vi "DisplayLeg.vi"(4 "Init?":bool, 6 "ClosePt":dbl[](array[numeric]), 7 "Field Force":dbl[](array[numeric]), 8 "AnkleTraj":dbl[][](array[numeric]), 9 "CablePos":cluster{"PointInGCS":dbl[][]}[](array[cluster]), 10 "Joint Coord in GCS":dbl[][](array[numeric]), 11 "3D graph in":refnum<k7>) -> (3 "3D graph out":refnum<k7>)   [LabVIEW 2014]
uses:
  <vilib>/Platform/NI_3dgraph.lvlib
  <vilib>/ptbypt/NI_PtbyPt.lvlib
panel:
  in  "sample length":i32=100
  out "LastPlotNum":i32=1
  out "error out":errorcluster
  in  "error in (no error)":errorcluster
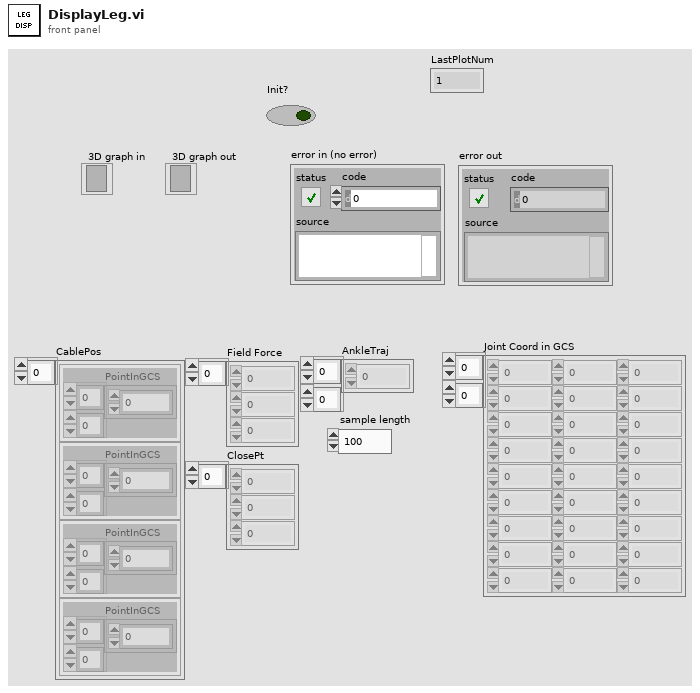
[diagram p1: front panel]
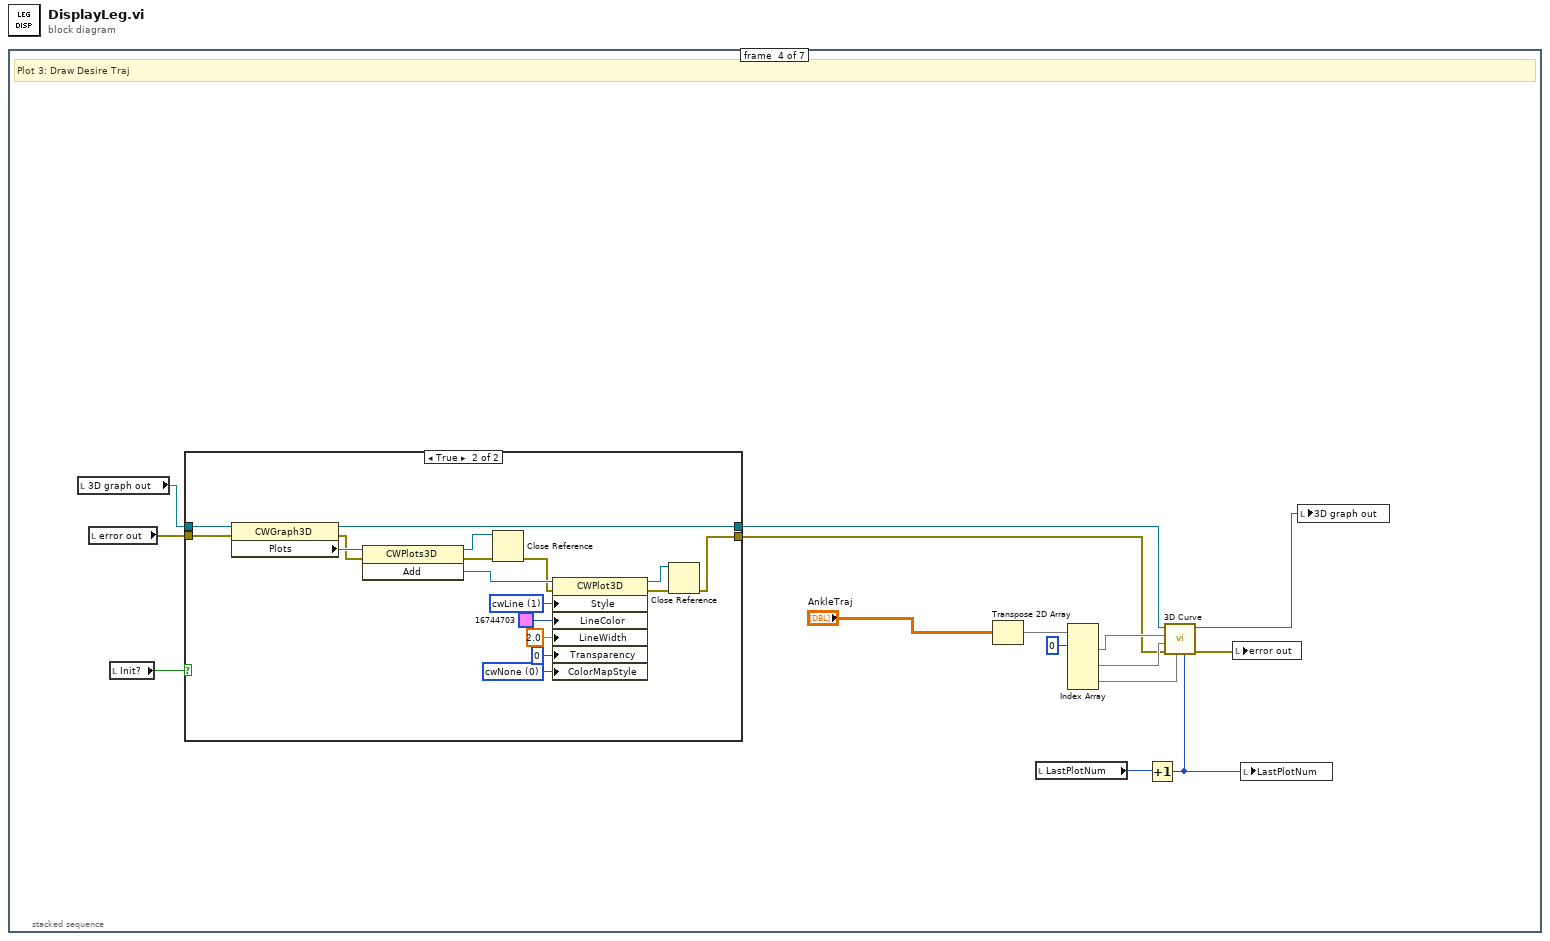
[diagram p0: block diagram]
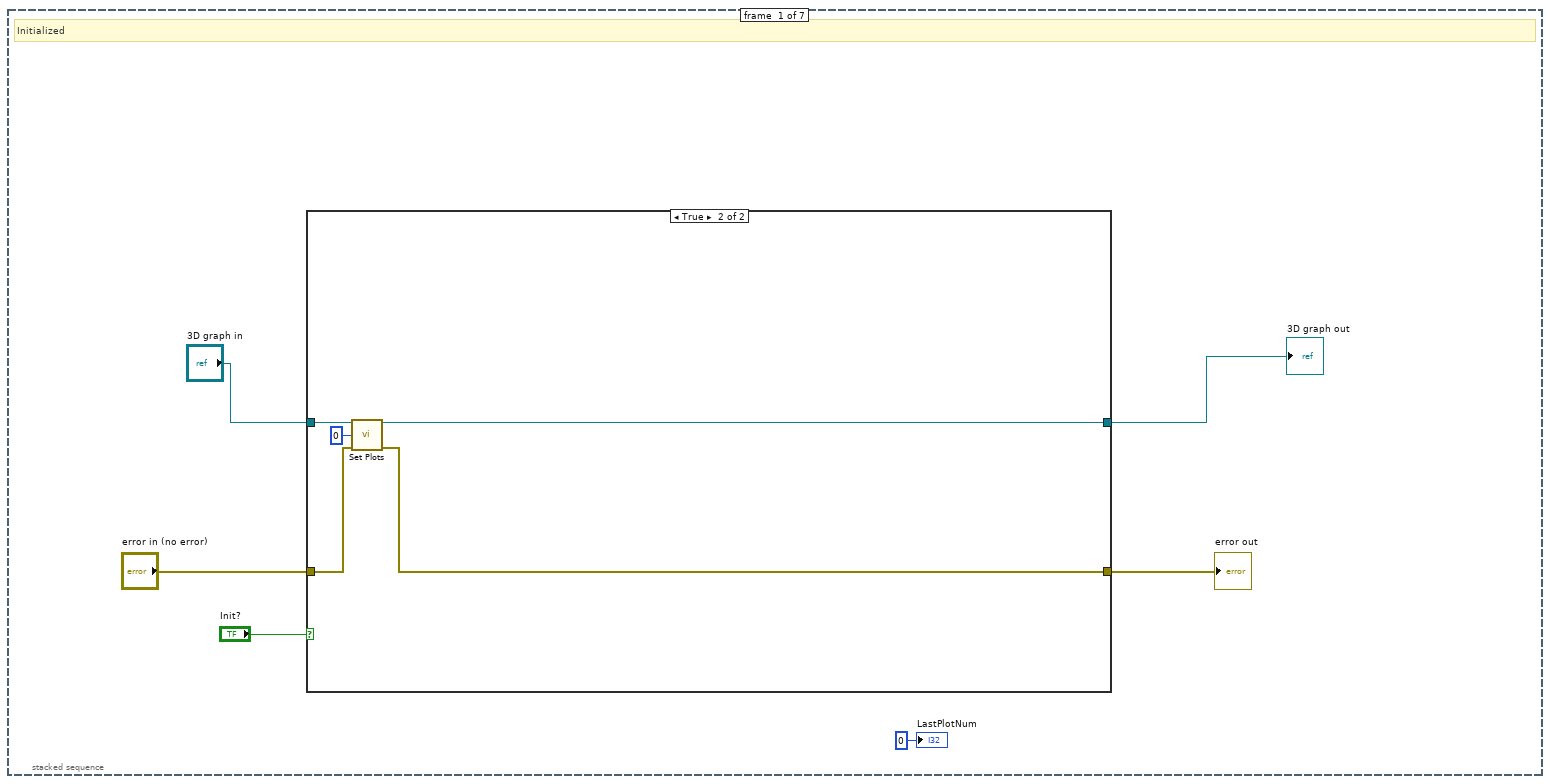
[diagram p2: hidden frame]
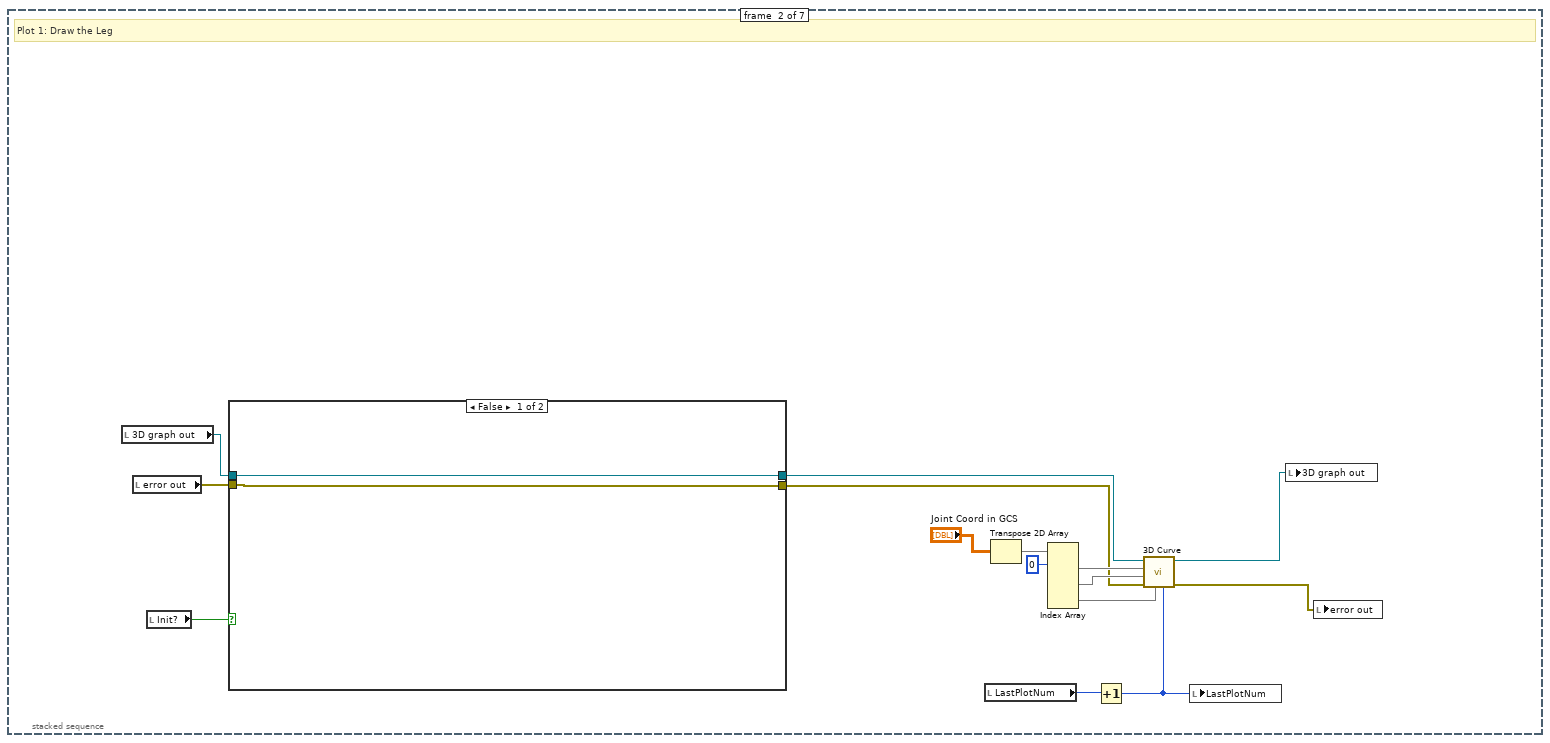
[diagram p4: hidden frame]
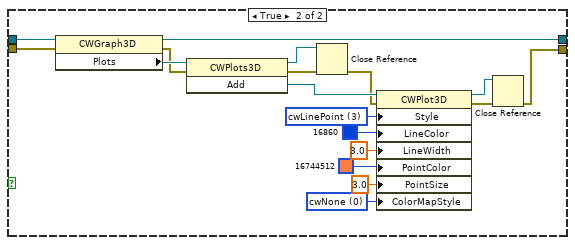
[diagram p5: hidden frame]
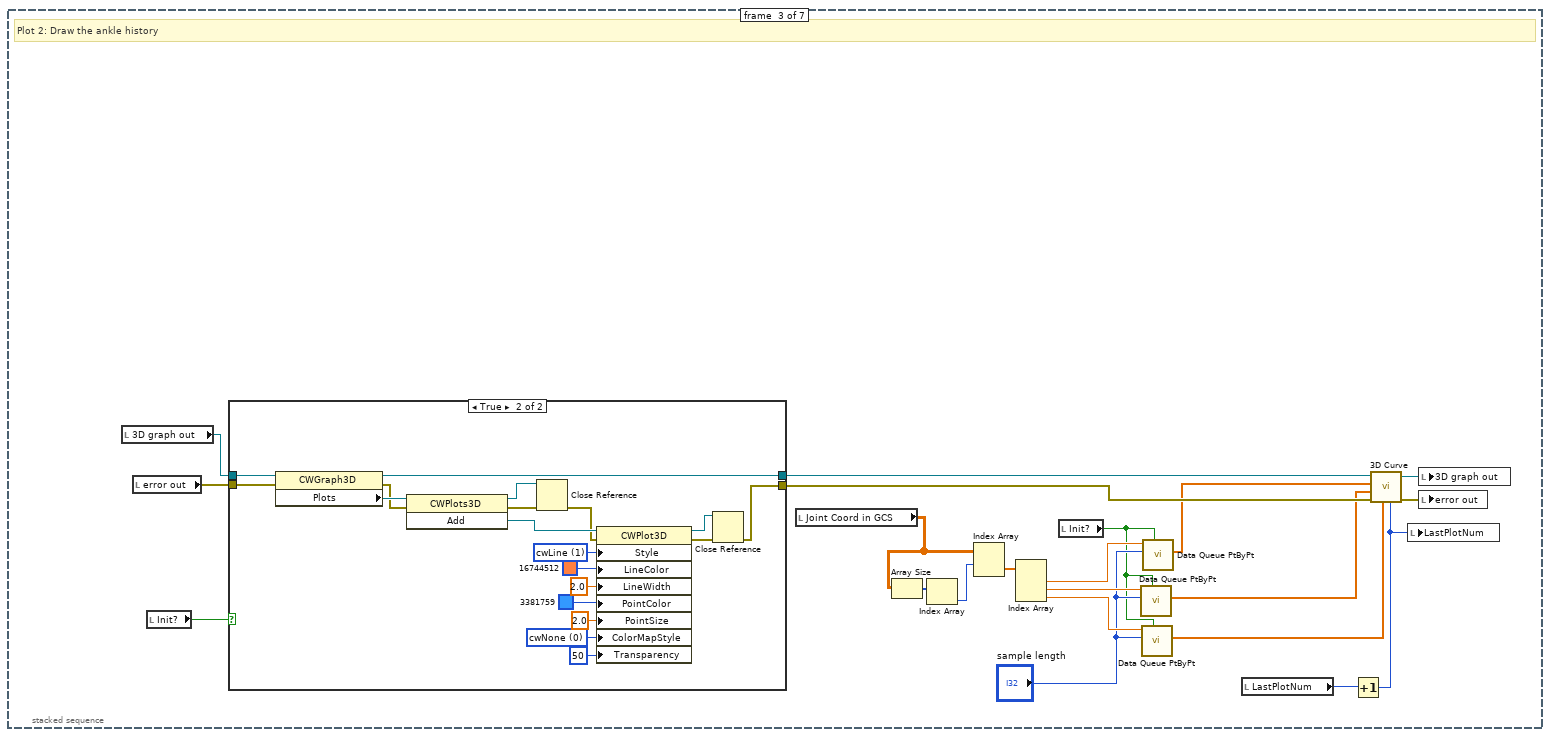
[diagram p6: hidden frame]
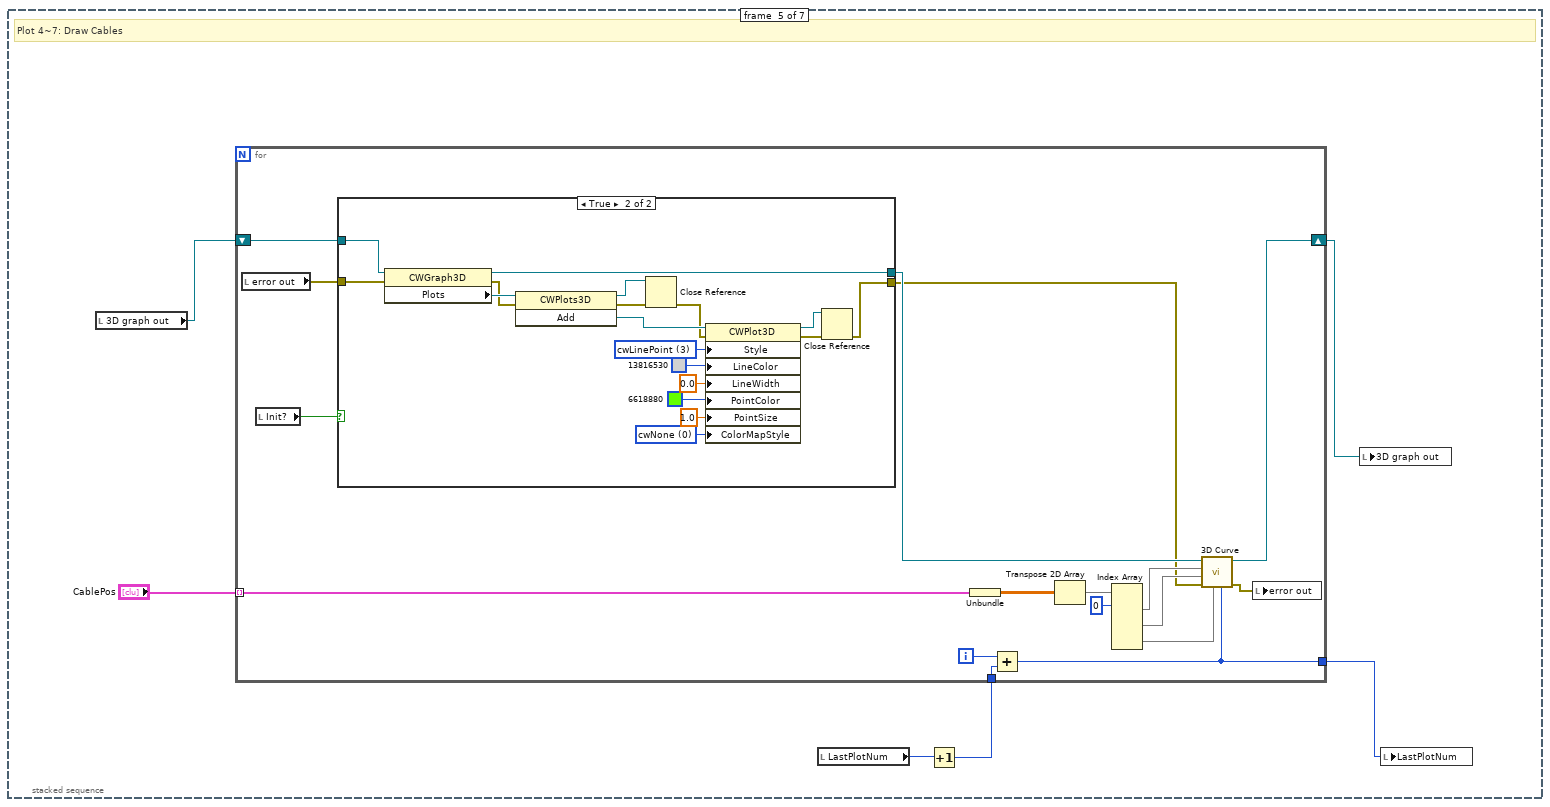
[diagram p9: hidden frame]
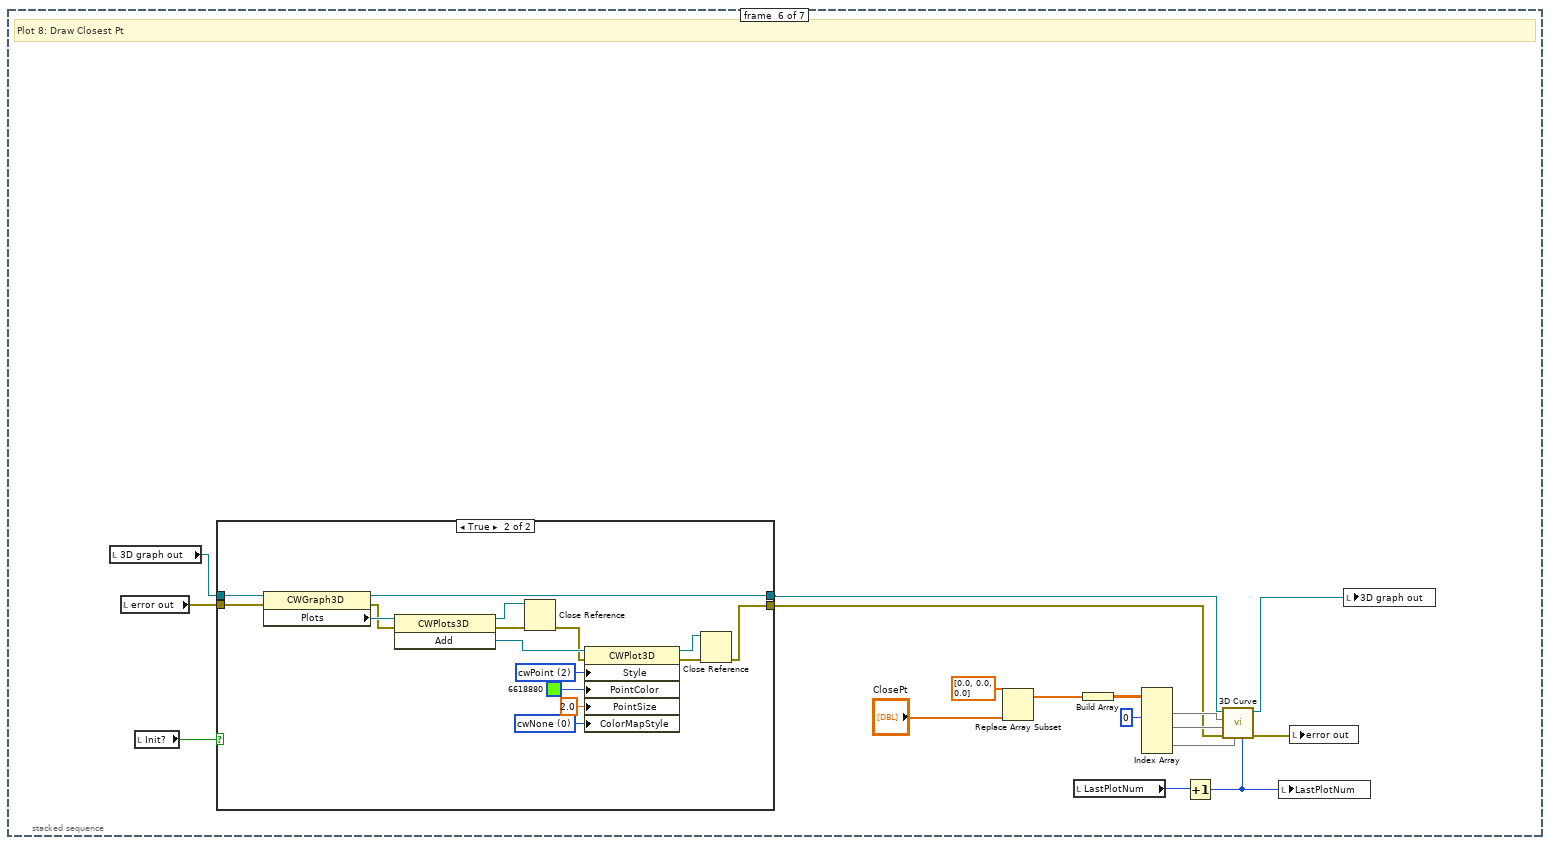
[diagram p11: hidden frame]
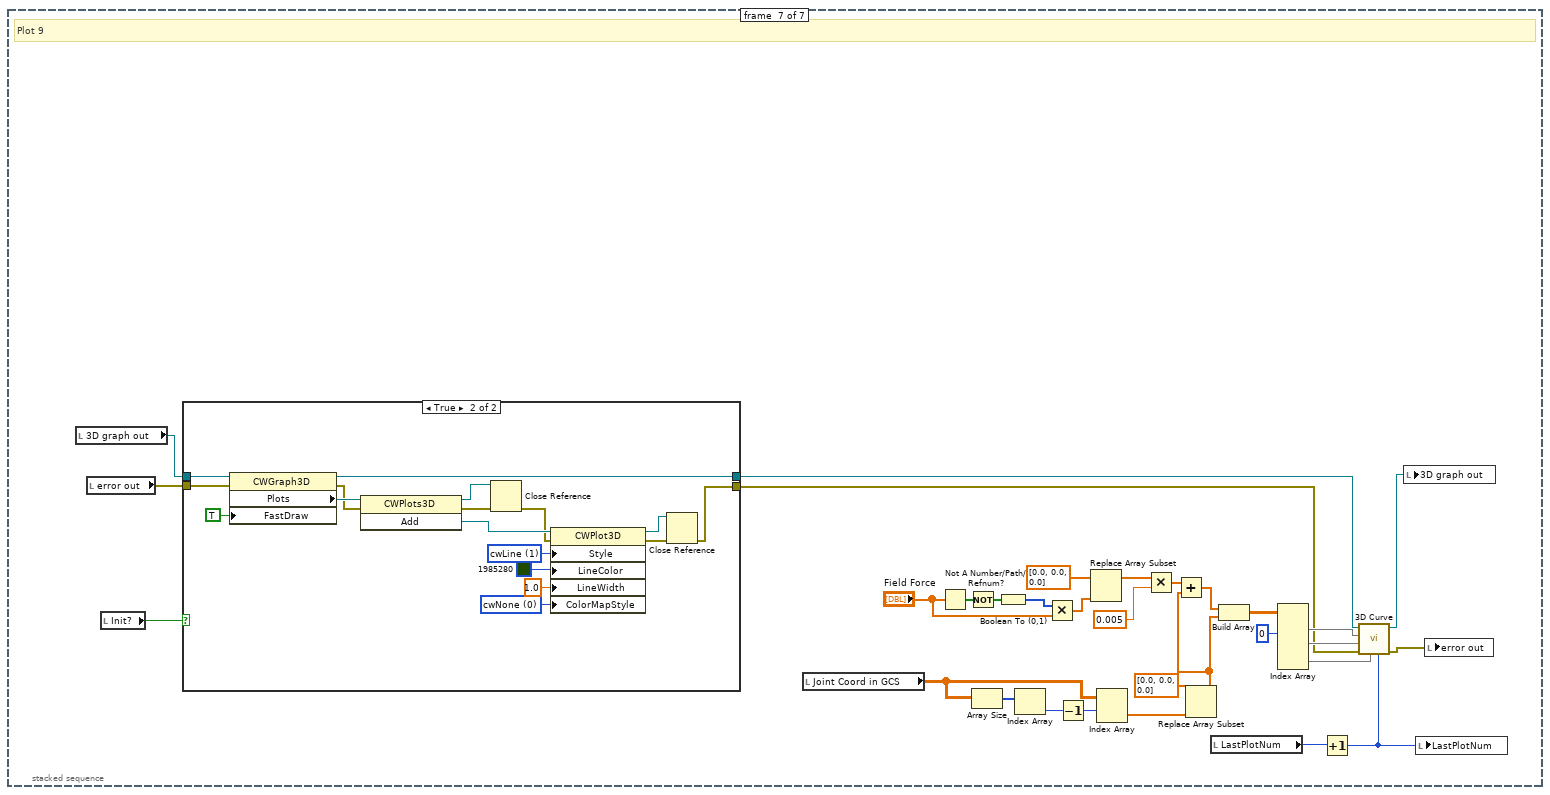
[diagram p13: hidden frame]
diagram:
  n1 = stacked-sequence {
    frame #0 {
      # "Initialized"
      n2 = case shown="True" "Init?" {
        tunnel: "3D graph in" -> [w8 w13]
        tunnel: [w8 w9] -> w5
        tunnel: [w7 w11] -> w3
        tunnel: "error in (no error)" -> [w7 w10]
        frame False {
        }
        frame True {
          n3 = call <vilib>:"Set Plots.vi"("3D graph"=w13, "# of plots(1)"=0, "error in (no error)"=w10) -> ("3D graph out"=w9:refnum<k7>, "error out"=w11:errorcluster)  [unwired: 11 in]
        }
      }
      "3D graph out" <- w5
      "error out" <- w3
      "LastPlotNum" <- 0 ("LastPlotNum 2")
    }
    frame #1 {
      # "Plot 1: Draw the Leg"
      n4 = local read "3D graph out"() -> (w20:refnum<k7>)
      n5 = local read "error out"() -> (w21:errorcluster)
      n6 = local read "Init?"() -> (w14:bool)
      n7 = case shown="False" w14 {
        tunnel: w21 -> [w29 w39]
        tunnel: w20 -> [w30 w34]
        tunnel: [w30 w33] -> w19
        tunnel: [w29 w32] -> w18
        frame False {
        }
        frame True {
          w31 = 0 items=["cwNone", "cwShaded", "cwColorSpectrum", "cwGrayScale", "cwCustom"] ("ColorMapStyle")
          w48 = 3 items=["cwLine"=1, "cwPoint"=2, "cwLinePoint"=3, "cwHiddenLine"=4, "cwSurface"=5, "cwSurfaceLine"=6, "cwSurfaceNormal"=7, "cwContourLine"=8, "cwSurfaceContour"=9] ("Style")
          n8 = property class="CWGraph3D"(reference=w34, error in=w39) -> (reference out=w33:refnum<k7>, error out=w45:errorcluster, "Plots"=w46:refnum<k7>)
          n9 = invoke class="CWPlots3D" method="Add"(reference=w46, error in=w45) -> (reference out=w44:refnum<k7>, error out=w43:errorcluster, "Add"=w47:refnum<k7>)  [unwired: 1 in]
          n10 = Close Reference(reference=w44, error in (no error)=w43) -> (error out=w42:errorcluster)
          n11 = property class="CWPlot3D"(reference=w47, error in=w42, "Style"=w48, "LineColor"=u32 16860, "LineWidth"=3.0, "PointColor"=u32 16744512, "PointSize"=3.0 ("LineWidth"), "ColorMapStyle"=w31) -> (reference out=w40:refnum<k7>, error out=w41:errorcluster)
          n12 = Close Reference(reference=w40, error in (no error)=w41) -> (error out=w32:errorcluster)
        }
      }
      n13 = local read "LastPlotNum"() -> (w16:i32)
      n14 = Transpose 2D Array(2D array="Joint Coord in GCS") -> (transposed array=w23:dbl[][])
      n15 = Index Array(array=w23, index (row) #1=0 ("index (row)")) -> (element #1=w25:dbl[], element #2=w26:dbl[], element #3=w27:dbl[])  [unwired: 5 in]
      n16 = Increment(x=w16) -> (x+1=w15:i32)
      n17 = call <vilib>:"3D Curve.vi"("plot number (1)"=w15, "z vector"=w27, "error in (no error)"=w18, "y vector"=w26, "x vector"=w25, "3D graph"=w19) -> ("error out"=w17:errorcluster, "3D graph out"=w22:refnum<k7>)  [unwired: 4 in]
      n18 = local write "LastPlotNum"(w15) -> ()
      n19 = local write "3D graph out"(w22) -> ()
      n20 = local write "error out"(w17) -> ()
    }
    frame #2 {
      # "Plot 2: Draw the ankle history"
      n21 = local read "3D graph out"() -> (w67:refnum<k7>)
      n22 = local read "error out"() -> (w68:errorcluster)
      n23 = local read "Init?"() -> (w61:bool)
      n24 = case shown="True" w61 {
        tunnel: w68 -> [w70 w81]
        tunnel: w67 -> [w71 w76]
        tunnel: [w71 w75] -> w66
        tunnel: [w70 w74] -> w65
        frame False {
        }
        frame True {
          w73 = 0 items=["cwNone", "cwShaded", "cwColorSpectrum", "cwGrayScale", "cwCustom"] ("ColorMapStyle")
          w90 = 1 items=["cwLine"=1, "cwPoint"=2, "cwLinePoint"=3, "cwHiddenLine"=4, "cwSurface"=5, "cwSurfaceLine"=6, "cwSurfaceNormal"=7, "cwContourLine"=8, "cwSurfaceContour"=9] ("Style")
          n25 = property class="CWGraph3D"(reference=w76, error in=w81) -> (reference out=w75:refnum<k7>, error out=w87:errorcluster, "Plots"=w88:refnum<k7>)
          n26 = invoke class="CWPlots3D" method="Add"(reference=w88, error in=w87) -> (reference out=w86:refnum<k7>, error out=w85:errorcluster, "Add"=w89:refnum<k7>)  [unwired: 1 in]
          n27 = Close Reference(reference=w86, error in (no error)=w85) -> (error out=w84:errorcluster)
          n28 = property class="CWPlot3D"(reference=w89, error in=w84, "Style"=w90, "LineColor"=u32 16744512, "LineWidth"=2.0, "PointColor"=u32 3381759, "PointSize"=2.0 ("LineWidth"), "ColorMapStyle"=w73, "Transparency"=50) -> (reference out=w82:refnum<k7>, error out=w83:errorcluster)
          n29 = Close Reference(reference=w82, error in (no error)=w83) -> (error out=w74:errorcluster)
        }
      }
      n30 = local read "Joint Coord in GCS"() -> (w58:dbl[][])
      n31 = Array Size(array=w58) -> (size(s)=w60:i32[])
      n32 = Index Array(array=w60) -> (element=w59:i32)  [unwired: 1 in]
      n33 = Index Array(array=w58, index (row)=w59) -> (element=w57:dbl[])  [unwired: 1 in]
      n34 = Index Array(array=w57) -> (element #1=w54:dbl, element #2=w55:dbl, element #3=w56:dbl)  [unwired: 3 in]
      n35 = local read "Init?"() -> (w49:bool)
      n36 = call <vilib>:"Data Queue PtByPt.vi"("initialize"=w49, "sample length"="sample length", "input data point"=w55) -> ("Current Queue"=w51:dbl[])  [unwired: 4 in, 4 out]
      n37 = call <vilib>:"Data Queue PtByPt.vi"("initialize"=w49, "sample length"="sample length", "input data point"=w56) -> ("Current Queue"=w50:dbl[])  [unwired: 4 in, 4 out]
      n38 = call <vilib>:"Data Queue PtByPt.vi"("initialize"=w49, "sample length"="sample length", "input data point"=w54) -> ("Current Queue"=w52:dbl[])  [unwired: 4 in, 4 out]
      n39 = local read "LastPlotNum"() -> (w63:i32)
      n40 = Increment(x=w63) -> (x+1=w62:i32)
      n41 = call <vilib>:"3D Curve.vi"("plot number (1)"=w62, "z vector"=w50, "error in (no error)"=w65, "y vector"=w51, "x vector"=w52, "3D graph"=w66) -> ("error out"=w64:errorcluster, "3D graph out"=w69:refnum<k7>)  [unwired: 4 in]
      n42 = local write "LastPlotNum"(w62) -> ()
      n43 = local write "3D graph out"(w69) -> ()
      n44 = local write "error out"(w64) -> ()
    }
    frame #3 {
      # "Plot 3: Draw Desire Traj"
      n45 = local read "3D graph out"() -> (w97:refnum<k7>)
      n46 = local read "error out"() -> (w98:errorcluster)
      n47 = local read "Init?"() -> (w93:bool)
      n48 = case shown="True" w93 {
        tunnel: w98 -> [w106 w115]
        tunnel: w97 -> [w107 w112]
        tunnel: [w107 w111] -> w96
        tunnel: [w106 w110] -> w92
        frame False {
        }
        frame True {
          w108 = 0 items=["cwNone", "cwShaded", "cwColorSpectrum", "cwGrayScale", "cwCustom"] ("ColorMapStyle")
          w124 = 1 items=["cwLine"=1, "cwPoint"=2, "cwLinePoint"=3, "cwHiddenLine"=4, "cwSurface"=5, "cwSurfaceLine"=6, "cwSurfaceNormal"=7, "cwContourLine"=8, "cwSurfaceContour"=9] ("Style")
          n49 = property class="CWGraph3D"(reference=w112, error in=w115) -> (reference out=w111:refnum<k7>, error out=w121:errorcluster, "Plots"=w122:refnum<k7>)
          n50 = invoke class="CWPlots3D" method="Add"(reference=w122, error in=w121) -> (reference out=w120:refnum<k7>, error out=w119:errorcluster, "Add"=w123:refnum<k7>)  [unwired: 1 in]
          n51 = Close Reference(reference=w120, error in (no error)=w119) -> (error out=w118:errorcluster)
          n52 = property class="CWPlot3D"(reference=w123, error in=w118, "Style"=w124, "LineColor"=u32 16744703, "LineWidth"=2.0, "Transparency"=0, "ColorMapStyle"=w108) -> (reference out=w116:refnum<k7>, error out=w117:errorcluster)
          n53 = Close Reference(reference=w116, error in (no error)=w117) -> (error out=w110:errorcluster)
        }
      }
      n54 = Transpose 2D Array(2D array="AnkleTraj") -> (transposed array=w100:dbl[][])
      n55 = local read "LastPlotNum"() -> (w95:i32)
      n56 = Index Array(array=w100, index (row) #1=0 ("index (row)")) -> (element #1=w102:dbl[], element #2=w103:dbl[], element #3=w104:dbl[])  [unwired: 5 in]
      n57 = Increment(x=w95) -> (x+1=w94:i32)
      n58 = call <vilib>:"3D Curve.vi"("plot number (1)"=w94, "z vector"=w104, "error in (no error)"=w92, "y vector"=w103, "x vector"=w102, "3D graph"=w96) -> ("error out"=w91:errorcluster, "3D graph out"=w99:refnum<k7>)  [unwired: 4 in]
      n59 = local write "error out"(w91) -> ()
      n60 = local write "LastPlotNum"(w94) -> ()
      n61 = local write "3D graph out"(w99) -> ()
    }
    frame #4 {
      # "Plot 4~7: Draw Cables"
      n62 = local read "3D graph out"() -> (w127:refnum<k7>)
      n63 = local read "LastPlotNum"() -> (w128:i32)
      n64 = Increment(x=w128) -> (x+1=w126:i32)
      n65 = for {
        tunnel: "CablePos" -> [w145] mode=indexing
        shift-right: [w143] -> w129
        shift-left: w127 -> [w136]
        tunnel: w126 -> [w134]
        tunnel: [w133] -> w125
        i -> [w139]
        n66 = local read "error out"() -> (w138:errorcluster)
        n67 = local read "Init?"() -> (w137:bool)
        n68 = case shown="True" w137 {
          tunnel: w138 -> [w149 w158]
          tunnel: [w148 w153] -> w135
          tunnel: [w149 w152] -> w132
          tunnel: w136 -> [w148 w150]
          frame False {
          }
          frame True {
            w151 = 0 items=["cwNone", "cwShaded", "cwColorSpectrum", "cwGrayScale", "cwCustom"] ("ColorMapStyle")
            w167 = 3 items=["cwLine"=1, "cwPoint"=2, "cwLinePoint"=3, "cwHiddenLine"=4, "cwSurface"=5, "cwSurfaceLine"=6, "cwSurfaceNormal"=7, "cwContourLine"=8, "cwSurfaceContour"=9] ("Style")
            n69 = property class="CWGraph3D"(reference=w150, error in=w158) -> (reference out=w153:refnum<k7>, error out=w164:errorcluster, "Plots"=w165:refnum<k7>)
            n70 = invoke class="CWPlots3D" method="Add"(reference=w165, error in=w164) -> (reference out=w163:refnum<k7>, error out=w162:errorcluster, "Add"=w166:refnum<k7>)  [unwired: 1 in]
            n71 = Close Reference(reference=w163, error in (no error)=w162) -> (error out=w161:errorcluster)
            n72 = property class="CWPlot3D"(reference=w166, error in=w161, "Style"=w167, "LineColor"=u32 13816530, "LineWidth"=0.0, "PointColor"=u32 6618880, "PointSize"=1.0 ("LineWidth"), "ColorMapStyle"=w151) -> (reference out=w159:refnum<k7>, error out=w160:errorcluster)
            n73 = Close Reference(reference=w159, error in (no error)=w160) -> (error out=w152:errorcluster)
          }
        }
        n74 = Unbundle(w145) -> ("PointInGCS"=w144:dbl[][])
        n75 = Add(x=w139, y=w134) -> (x+y=w133:i32)
        n76 = Transpose 2D Array(2D array=w144) -> (transposed array=w146:dbl[][])
        n77 = Index Array(array=w146, index (row) #1=0 ("index (row)")) -> (element #1=w142:dbl[], element #2=w141:dbl[], element #3=w140:dbl[])  [unwired: 5 in]
        n78 = call <vilib>:"3D Curve.vi"("plot number (1)"=w133, "z vector"=w140, "error in (no error)"=w132, "y vector"=w141, "x vector"=w142, "3D graph"=w135) -> ("error out"=w131:errorcluster, "3D graph out"=w143:refnum<k7>)  [unwired: 4 in]
        n79 = local write "error out"(w131) -> ()
      }
      n80 = local write "3D graph out"(w129) -> ()
      n81 = local write "LastPlotNum"(w125) -> ()
    }
    frame #5 {
      # "Plot 8: Draw Closest Pt"
      n82 = local read "3D graph out"() -> (w174:refnum<k7>)
      n83 = local read "error out"() -> (w175:errorcluster)
      n84 = local read "Init?"() -> (w173:bool)
      n85 = case shown="True" w173 {
        tunnel: w175 -> [w185 w193]
        tunnel: w174 -> [w186 w190]
        tunnel: [w186 w189] -> w172
        tunnel: [w185 w188] -> w169
        frame False {
        }
        frame True {
          w187 = 0 items=["cwNone", "cwShaded", "cwColorSpectrum", "cwGrayScale", "cwCustom"] ("ColorMapStyle")
          w202 = 2 items=["cwLine"=1, "cwPoint"=2, "cwLinePoint"=3, "cwHiddenLine"=4, "cwSurface"=5, "cwSurfaceLine"=6, "cwSurfaceNormal"=7, "cwContourLine"=8, "cwSurfaceContour"=9] ("Style")
          n86 = property class="CWGraph3D"(reference=w190, error in=w193) -> (reference out=w189:refnum<k7>, error out=w199:errorcluster, "Plots"=w200:refnum<k7>)
          n87 = invoke class="CWPlots3D" method="Add"(reference=w200, error in=w199) -> (reference out=w198:refnum<k7>, error out=w197:errorcluster, "Add"=w201:refnum<k7>)  [unwired: 1 in]
          n88 = Close Reference(reference=w198, error in (no error)=w197) -> (error out=w196:errorcluster)
          n89 = property class="CWPlot3D"(reference=w201, error in=w196, "Style"=w202, "PointColor"=u32 6618880, "PointSize"=2.0 ("LineWidth"), "ColorMapStyle"=w187) -> (reference out=w194:refnum<k7>, error out=w195:errorcluster)
          n90 = Close Reference(reference=w194, error in (no error)=w195) -> (error out=w188:errorcluster)
        }
      }
      n91 = Replace Array Subset(array=dbl[] [0.0, 0.0, 0.0], new element="ClosePt") -> (w182:dbl[])  [unwired: 1 in]
      n92 = local read "LastPlotNum"() -> (w171:i32)
      n93 = Build Array(w182) -> (w181:dbl[][])
      n94 = Index Array(array=w181, index (col) #1=0 ("disabled index (col)")) -> (element #1=w179:dbl[], element #2=w178:dbl[], element #3=w177:dbl[])  [unwired: 5 in]
      n95 = Increment(x=w171) -> (x+1=w170:i32)
      n96 = call <vilib>:"3D Curve.vi"("plot number (1)"=w170, "z vector"=w177, "error in (no error)"=w169, "y vector"=w178, "x vector"=w179, "3D graph"=w172) -> ("error out"=w168:errorcluster, "3D graph out"=w176:refnum<k7>)  [unwired: 4 in]
      n97 = local write "LastPlotNum"(w170) -> ()
      n98 = local write "error out"(w168) -> ()
      n99 = local write "3D graph out"(w176) -> ()
    }
    frame #6 {
      # "Plot 9"
      n100 = local read "3D graph out"() -> (w209:refnum<k7>)
      n101 = local read "error out"() -> (w210:errorcluster)
      n102 = local read "Init?"() -> (w208:bool)
      n103 = case shown="True" w208 {
        tunnel: w210 -> [w234 w243]
        tunnel: w209 -> [w235 w240]
        tunnel: [w235 w239] -> w207
        tunnel: [w234 w238] -> w204
        frame False {
        }
        frame True {
          w237 = 0 items=["cwNone", "cwShaded", "cwColorSpectrum", "cwGrayScale", "cwCustom"] ("ColorMapStyle")
          w252 = 1 items=["cwLine"=1, "cwPoint"=2, "cwLinePoint"=3, "cwHiddenLine"=4, "cwSurface"=5, "cwSurfaceLine"=6, "cwSurfaceNormal"=7, "cwContourLine"=8, "cwSurfaceContour"=9] ("Style")
          n104 = property class="CWGraph3D"(reference=w240, error in=w243, "FastDraw"=TRUE) -> (reference out=w239:refnum<k7>, error out=w249:errorcluster, "Plots"=w250:refnum<k7>)
          n105 = invoke class="CWPlots3D" method="Add"(reference=w250, error in=w249) -> (reference out=w248:refnum<k7>, error out=w247:errorcluster, "Add"=w251:refnum<k7>)  [unwired: 1 in]
          n106 = Close Reference(reference=w248, error in (no error)=w247) -> (error out=w246:errorcluster)
          n107 = property class="CWPlot3D"(reference=w251, error in=w246, "Style"=w252, "LineColor"=u32 1985280, "LineWidth"=1.0, "ColorMapStyle"=w237) -> (reference out=w244:refnum<k7>, error out=w245:errorcluster)
          n108 = Close Reference(reference=w244, error in (no error)=w245) -> (error out=w238:errorcluster)
        }
      }
      n109 = local read "Joint Coord in GCS"() -> (w233:dbl[][])
      n110 = Not A Number/Path/Refnum?(number/path/refnum="Field Force") -> (NaN/Path/Refnum?=w216:bool[])
      n111 = Not(x=w216) -> (.not. x?=w215:bool[])
      n112 = Array Size(array=w233) -> (size(s)=w222:i32[])
      n113 = Boolean To (0,1)(Boolean=w215) -> (0, 1=w214:i16[])
      n114 = Index Array(array=w222) -> (element=w224:i32)  [unwired: 1 in]
      n115 = Multiply(x=w214, y="Field Force") -> (x*y=w212:dbl[])
      n116 = Decrement(x=w224) -> (x-1=w223:i32)
      n117 = Replace Array Subset(array=dbl[] [0.0, 0.0, 0.0], new element=w212) -> (w229:dbl[])  [unwired: 1 in]
      n118 = Index Array(array=w233, index (row)=w223) -> (element=w231:dbl[])  [unwired: 1 in]
      n119 = Multiply(x=w229, y=0.005) -> (x*y=w221:dbl[])
      n120 = Replace Array Subset(array=dbl[] [0.0, 0.0, 0.0], new element=w231) -> (w232:dbl[])  [unwired: 1 in]
      n121 = Add(x=w221, y=w232) -> (x+y=w218:dbl[])
      n122 = local read "LastPlotNum"() -> (w206:i32)
      n123 = Build Array(w218, w232) -> (w219:dbl[][])
      n124 = Index Array(array=w219, index (col) #1=0 ("disabled index (col)")) -> (element #1=w225:dbl[], element #2=w226:dbl[], element #3=w227:dbl[])  [unwired: 5 in]
      n125 = Increment(x=w206) -> (x+1=w205:i32)
      n126 = call <vilib>:"3D Curve.vi"("plot number (1)"=w205, "z vector"=w227, "error in (no error)"=w204, "y vector"=w226, "x vector"=w225, "3D graph"=w207) -> ("error out"=w203:errorcluster, "3D graph out"=w211:refnum<k7>)  [unwired: 4 in]
      n127 = local write "3D graph out"(w211) -> ()
      n128 = local write "LastPlotNum"(w205) -> ()
      n129 = local write "error out"(w203) -> ()
    }
  }
